vi "AKD Get MT Active.vi"(0 "TCP Refnum in":refnum<k5>, 11 "error in":errorcluster) -> (4 "TCP Refnum out":refnum<k5>, 6 "MT active?":bool, 8 "Holding Registers":u16[](array[numeric]), 15 "error out":errorcluster)   [LabVIEW 2019]
doc: "This VI will read the drive motion status and provide a flag to indicate whether a Motion Task is currently active (True) or not (False)"
uses:
  MODBUS/NI Modbus.llb/MB Ethernet Master Query Read Holding Registers (poly).vi
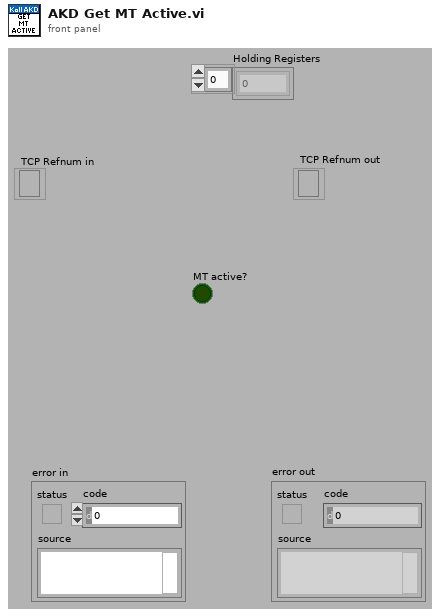
[diagram p1: front panel]
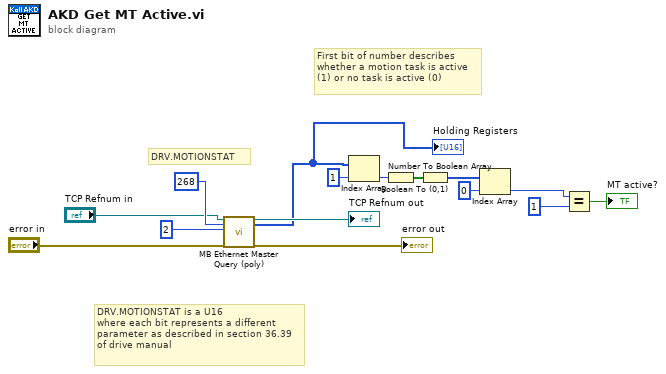
[diagram p0: block diagram]
diagram:
  # "First bit of number describes\nwhether a motion task is active\n(1) or no task is active (0)"
  # "DRV.MOTIONSTAT is a U16 \nwhere each bit represents a different \nparameter as described in section 36.39\nof drive manual"
  # "DRV.MOTIONSTAT"
  n1 = call-poly "MB Ethernet Master Query (poly).vi"("TCP Connection Refnum in"="TCP Refnum in", "Starting Address"=u16 268, "Quantity"=u16 2, "error in"="error in") -> ("TCP Connection Refnum (dup)"=→"TCP Refnum out":refnum<k5>, "Holding Registers"=w1:u16[], "error out"=→"error out":errorcluster)  [unwired: 12 in, 1 out]
  "Holding Registers" <- w1
  n2 = Index Array(array=w1, index=1) -> (element=w12:u16)
  n3 = Number To Boolean Array(number=w12) -> (Boolean array=w11:bool[])
  n4 = Boolean To (0,1)(Boolean=w11) -> (0, 1=w10:i16[])
  n5 = Index Array(array=w10, index=0) -> (element=w6:i16)
  n6 = Equal?(x=w6, y=i16 1) -> (x = y?=→"MT active?":bool)
